vi "BooleanToU8.vi"(1 "布尔":bool) -> (0 "U8":u8)   [LabVIEW 2012]
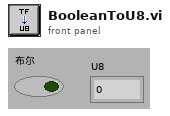
[diagram p1: front panel]
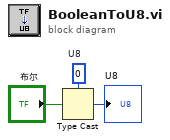
[diagram p0: block diagram]
diagram:
  w2 = u8 0  # U8
  n1 = Type Cast(type=w2, x="布尔") -> (*(type *) &x=→"U8":u8)
